vi "ClientCode.vi"(8 "error in (no error)":errorcluster, 10 "OrderPizza":T2, 11 "PizzaTestDrive in":refnum<class "PizzaTestDrive.lvclass">) -> (0 "error out":errorcluster, 3 "PizzaTestDrive out":refnum<class "PizzaTestDrive.lvclass">)   [LabVIEW 2020]
uses:
  PizzaStore/PizzaStore.lvclass
  Pizza/Pizza.lvclass
  PizzaTestDrive.lvclass
  OrderPizza.ctl
  PizzaStore/TypeDef/PizzaId.ctl
panel:
  in  "PizzaStoreList":refnum<class "PizzaStore.lvclass">[](array[class])
  in  "PizzaId":T1
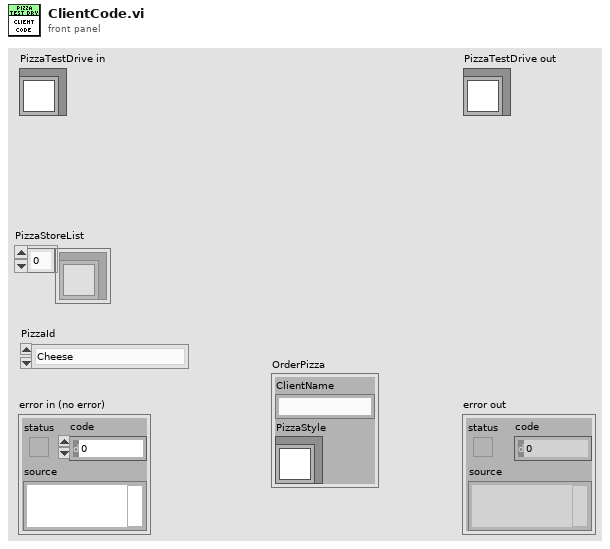
[diagram p1: front panel]
types:
  T1 = typedef "FactoryMethod.lvlib/PizzaFactoryMethod.lvlib/PizzaStore.lvclass/PizzaId.ctl" = enum16{"Cheese", "Clam", "Pepperoni", "Veggie"}
  T2 = typedef "OrderPizza.ctl" = cluster{"ClientName":string, "PizzaStyle":refnum<class "PizzaStore.lvclass">}
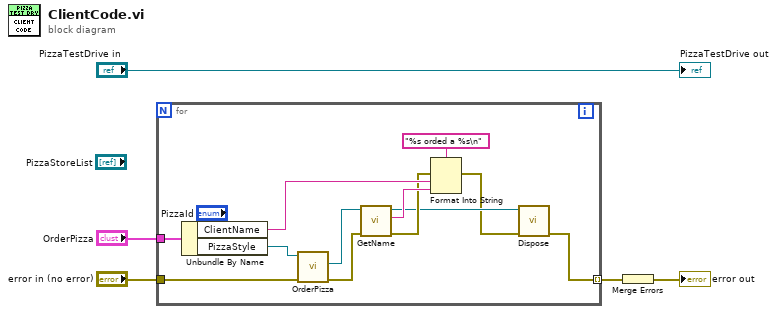
[diagram p0: block diagram]
diagram:
  n1 = for {
    tunnel: "OrderPizza" -> [w17]
    tunnel: [w6] -> w1 mode=indexing
    tunnel: "error in (no error)" -> [w9]
    n2 = Unbundle By Name(w17) -> ("ClientName"=w15:string, "PizzaStyle"=w16:refnum<class "PizzaStore.lvclass">)
    n3 = call "OrderPizza.vi"("error in (no error)"=w9, "PizzaStore"=w16) -> ("error out"=w11:errorcluster, "Pizza"=w14:refnum<class "Pizza.lvclass">)  [unwired: 7 in, 1 out]
    n4 = call "GetName.vi"("error in (no error)"=w11, "Pizza in"=w14) -> ("error out"=w12:errorcluster, "Name"=w13:string, "Pizza out"=w8:refnum<class "Pizza.lvclass">)  [unwired: 7 in]
    n5 = Format Into String(format string="%s orded a %s\n", error in=w12, w15, w13) -> (error out=w7:errorcluster)  [unwired: 1 in, 1 out]
    n6 = call-dynamic "Dispose.vi"("error in (no error)"=w7, "IDisposable"=w8) -> ("error out"=w6:errorcluster)  [unwired: 9 in]
  }
  n7 = Merge Errors(w1) -> (→"error out":errorcluster)
  "PizzaTestDrive out" <- "PizzaTestDrive in"
